vi "Q_limiter.vi"(10 "IN Q":dbl=750.0) -> (2 "OUT Q":dbl)   [LabVIEW 2021]
panel:
  out "In Range?":bool
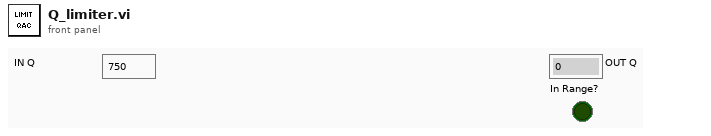
[diagram p1: front panel]
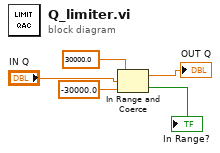
[diagram p0: block diagram]
diagram:
  n1 = In Range and Coerce(upper limit=30000.0 ("x"), x="IN Q", lower limit=-30000.0 ("x")) -> (coerced(x)=→"OUT Q":dbl, In Range?=→"In Range?":bool)
